vi "Get ROI Cords Im Index.vi"(0 "Image Idx":i32, 11 "Error In":errorcluster) -> (4 "H Offset":i32, 6 "V Offset":i32, 8 "H Width":i32, 10 "V Width":i32, 15 "Error Out":errorcluster)   [LabVIEW 2020]
uses:
  Display Module Custom Controls/ROI Descriptor.ctl
  <vilib>/vision/Image Controls.llb/IMAQ Image.ctl
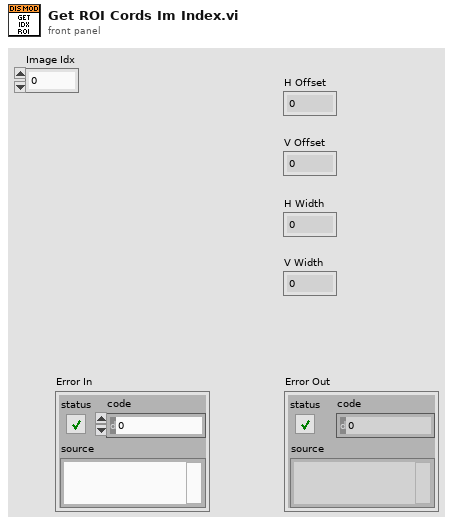
[diagram p1: front panel]
types:
  T1 = typedef "IMAQ Image.ctl" = refnum<image>
  T2 = typedef "ROI Descriptor.ctl" = cluster{"Global Rectangle":i32[], "Contours":cluster{"Contour Type":u32, "ROI Type":u32, "Points":i32[]}[]}
  T3 = typedef "Camera IMAQ Key Info.ctl" = cluster{"Frame":u32, "Sensor Height":i32, "Sensor Width":i32, "ROI Height":i32, "ROI Width":i32, "ROI Enable?":bool, "Bit per Pixel":u8}
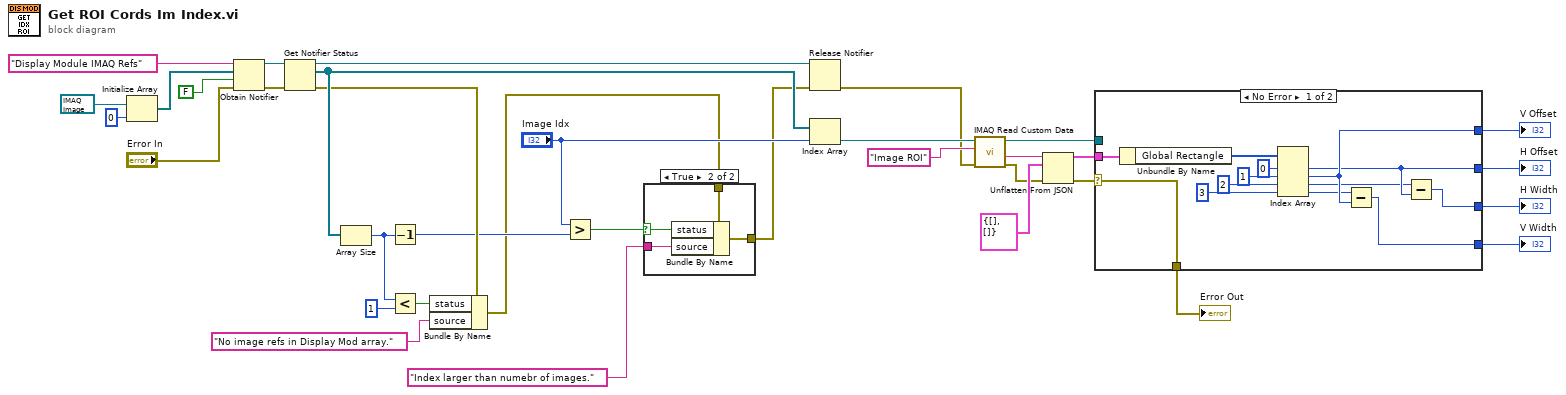
[diagram p0: block diagram]
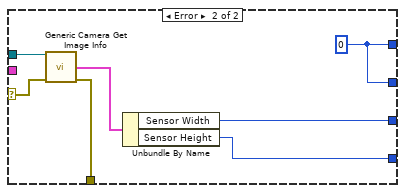
[diagram p3: hidden frame]
diagram:
  n1 = Initialize Array(T1 refnum ("New Image"), 0 ("dimension size")) -> (w19:T1[])
  n2 = Obtain Notifier(name (unnamed)="Display Module IMAQ Refs", notification data type=w19, create if not found? (T)=FALSE, error in (no error)="Error In") -> (notifier out=w18:refnum<notifier>, error out=w17:errorcluster)  [unwired: 1 out]
  n3 = Get Notifier Status(notifier=w18, error in (no error)=w17) -> (notifier out=w16:refnum<notifier>, current notification=w12:T1[], error out=w11:errorcluster)  [unwired: 2 out]
  n4 = Array Size(array=w12) -> (size(s)=w7:i32)
  n5 = Decrement(x=w7) -> (x-1=w6:i32)
  n6 = Less?(x=w7, y=1) -> (x < y?=w9:bool)
  n7 = Bundle By Name(cluster=w11, "status"=w9, "source"="No image refs in Display Mod array.") -> (w4:errorcluster)
  n8 = Greater?(x="Image Idx", y=w6) -> (0:w2:bool)
  n9 = case shown="True" w2 {
    selector: w2 -> [_ w38]
    tunnel: w4 -> [w36 w40]
    tunnel: "Index larger than numebr of images." ("source") -> [_ w39]
    tunnel: [w36 w37] -> w1
    frame False {
    }
    frame True {
      n10 = Bundle By Name(cluster=w40, "status"=w38, "source"=w39) -> (w37:errorcluster)
    }
  }
  n11 = Release Notifier(notifier=w16, error in (no error)=w1) -> (error out=w13:errorcluster)  [unwired: 1 in, 2 out]
  n12 = Index Array(array=w12, index="Image Idx") -> (element=w14:T1)
  n13 = call "IMAQ Read Custom Data"("error in (no error)"=w13, "Key"="Image ROI", "Image"=w14) -> ("error out"=w27:errorcluster, "Custom Data Out"=w28:string, "Image (duplicate)"=w30:T1)  [unwired: 6 in]
  n14 = Unflatten From JSON(JSON string=w28, type and defaults=T2 {"Global Rectangle"=[], "Contours"=[]} ("Image ROI Descriptor"), error in (no error)=w27) -> (value=w25:T2, error out=w26:errorcluster)  [unwired: 4 in]
  n15 = case shown="No Error" w26 {
    selector: w26 -> [w41 w54]
    tunnel: [w53 w56] -> w35
    tunnel: [w52 w56] -> w34
    tunnel: [w51 w58] -> w33
    tunnel: [w50 w57] -> w32
    tunnel: w30 -> [_ w60]
    tunnel: [w41 w55] -> w24
    tunnel: w25 -> [w42 _]
    frame No Error {
      n16 = Unbundle By Name(w42) -> ("Global Rectangle"=w49:i32[])
      n17 = Index Array(array=w49, index #1=0 ("index"), index #2=1 ("index"), index #3=2 ("index"), index #4=3 ("index")) -> (element #1=w52:i32, element #2=w53:i32, element #3=w43:i32, element #4=w44:i32)
      n18 = Subtract(x=w44, y=w53) -> (x-y=w51:i32)
      n19 = Subtract(x=w43, y=w52) -> (x-y=w50:i32)
    }
    frame Error {
      w56 = 0
      n20 = call "Generic Camera Get Image Info.vi"("Image Ref"=w60, "Error In"=w54) -> ("Camera Image Info"=w59:T3, "Error Out"=w55:errorcluster)  [unwired: 11 in, 1 out]
      n21 = Unbundle By Name(w59) -> ("Sensor Width"=w57:i32, "Sensor Height"=w58:i32)
    }
  }
  "V Offset" <- w35
  "V Width" <- w33
  "H Width" <- w32
  "H Offset" <- w34
  "Error Out" <- w24
